vi "Installer Pre-Uninstall Action.vi"   [LabVIEW 2015]
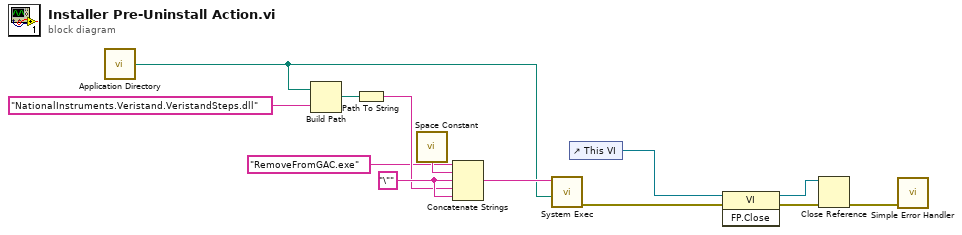
[diagram p0: block diagram]
diagram:
  w13 = "\"" ("string")
  n1 = call <vilib>:"Application Directory.vi"() -> ("Application Directory"=w6:path)
  n2 = Build Path(base path=w6, name or relative path="NationalInstruments.Veristand.VeristandSteps.dll" ("command line")) -> (appended path=w11:path)
  n3 = Path To String(path=w11) -> (string=w9:string)
  n4 = call <vilib>:"Space Constant.vi"() -> ("String"=w12:string)
  n5 = Concatenate Strings("RemoveFromGAC.exe" ("string"), w12, w13, w9, w13) -> (w7:string)
  n6 = call <vilib>:"System Exec.vi"("working directory"=w6, "command line"=w7) -> ("error out"=w1:errorcluster)  [unwired: 6 in, 3 out]
  n7 = control-ref of="This VI"() -> (w5:refnum<vi>)
  n8 = invoke class="VI" method="FP.Close"(reference=w5, error in=w1) -> (reference out=w3:refnum<vi>, error out=w4:errorcluster)  [unwired: 1 in, 1 out]
  n9 = Close Reference(reference=w3, error in (no error)=w4) -> (error out=w2:errorcluster)
  n10 = call <vilib>:"Simple Error Handler.vi"("error in (no error)"=w2) -> ()  [unwired: 4 in, 5 out]
